vi "measure_pulse_sweep.vi"(0 "Scan settings":T1={"Start voltage (V)"=0.0, "End voltage (V)"=1.4, "Number of steps"=10, "Settling delay (ms)"=10.0, "Dual sweep"=0, "Stabilisation time (s)"=0.0, "Stabilisation mode"=0, "Stabilisation value (V or A) "=0.0, "No. of repeat scans"=2.0, "Repeat scans"=0, "Logarithmic sweep"=0, "Electrode configuration"=0, "Sweep mode"=0, "Auto settling delay"=1, "Pulse off time (ms)"=0.0, "Integration time (ms)"=1.0, "Current range"=0, "Enable display"=0, "Enable concurrent measurements"=1, "Concurrent measurements"=1} {"Concurrent measurements" items=["Volts", "Current", "Resistance", "Volt, Current", "Volts, Resistance", "Current, Resistance", "All"]; "Enable concurrent measurements" items=["False", "True"]; "Enable display" items=["False", "True"]; "Current range" items=["Auto", "1 uA", "10 uA", "100 uA", "1 mA", "10 mA", "100 mA", "1 A"]; "Integration time (ms)" min=0.2 max=200.0; "Pulse off time (ms)" min=0.0; "Auto settling delay" items=["False", "True"]; "Sweep mode" items=["Staircase", "Pulsed"]; "Electrode configuration" items=["2-wire", "4-wire"]; "Logarithmic sweep" items=["False", "True"]; "Repeat scans" items=["False", "True"]; "No. of repeat scans" min=1.0 step=1.0; "Stabilisation mode" items=["V", "I"]; "Dual sweep" items=["False", "True"]; "Settling delay (ms)" min=0.0 max=999999.9}, 7 "Area (cm^2)":dbl, 9 "VISA Refnum in":refnum<visa-resource-name>="GPIB1::26::INSTR", 11 "Filename":path, 12 "Stabilisation filename":path) -> (6 "JV Curve":cluster{dbl[], dbl[]}(graph))   [LabVIEW 2016]
uses:
  TypeDefs/settings.ctl
  <instrlib>/Keithley 24XX/Public/Data/Read (Multiple Points).vi
  <vilib>/Utility/file.llb/Write Delimited Spreadsheet (DBL).vi
  <instrlib>/Keithley 24XX/Keithley 24XX.lvlib
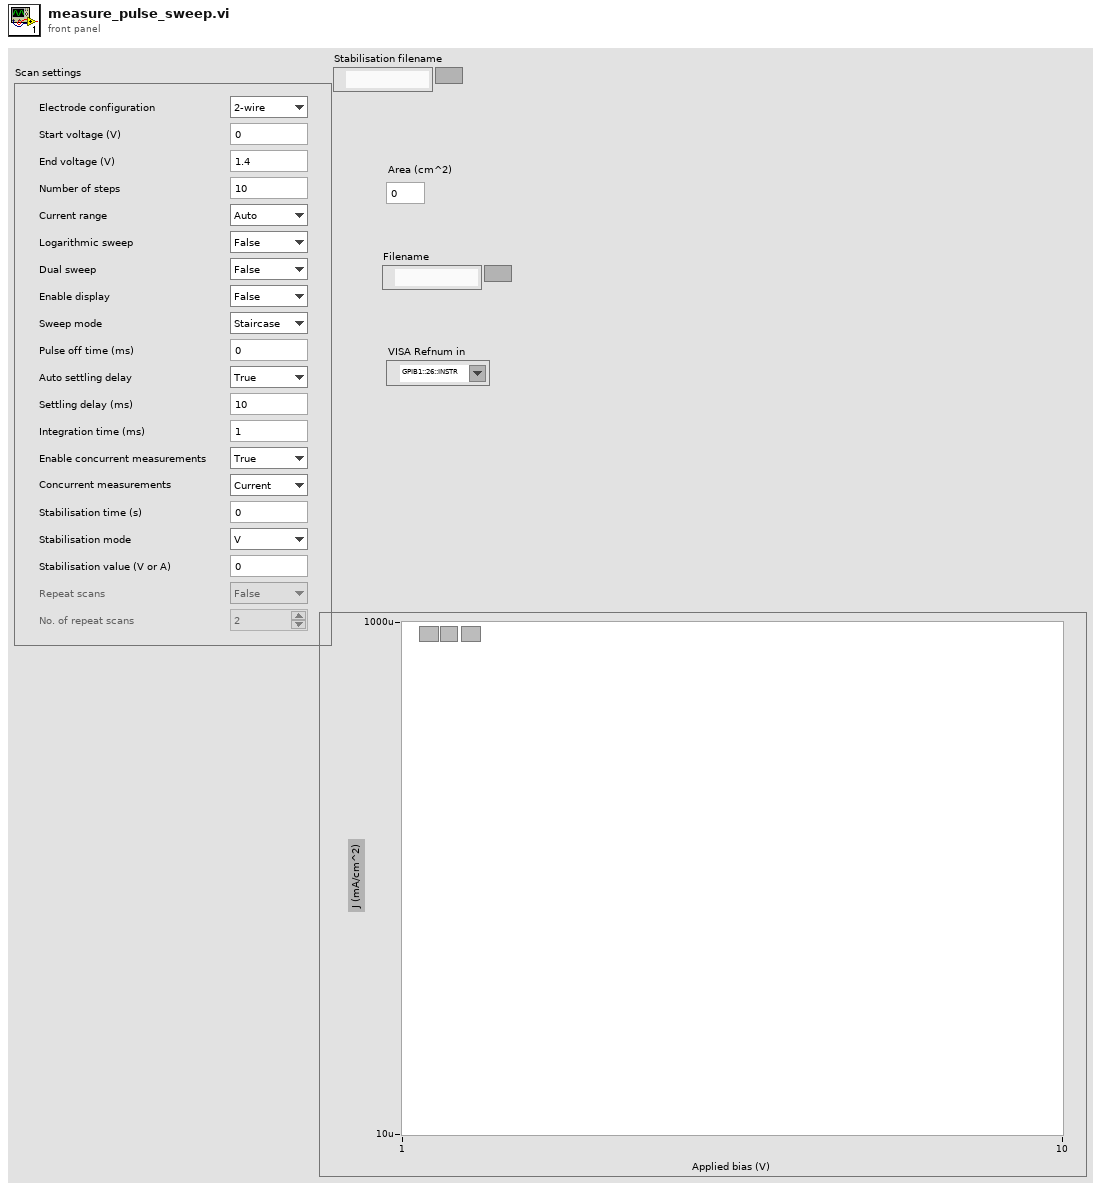
[diagram p1: front panel]
types:
  T1 = typedef "settings.ctl" = cluster{"Start voltage (V)":dbl, "End voltage (V)":dbl, "Number of steps":u32, "Settling delay (ms)":dbl, "Dual sweep":u16, "Stabilisation time (s)":dbl, "Stabilisation mode":u16, "Stabilisation value (V or A) ":dbl, "No. of repeat scans":dbl, "Repeat scans":u16, "Logarithmic sweep":u16, "Electrode configuration":u16, "Sweep mode":u16, "Auto settling delay":u16, "Pulse off time (ms)":dbl, "Integration time (ms)":dbl, "Current range":u16, "Enable display":u16, "Enable concurrent measurements":u16, "Concurrent measurements":u16}
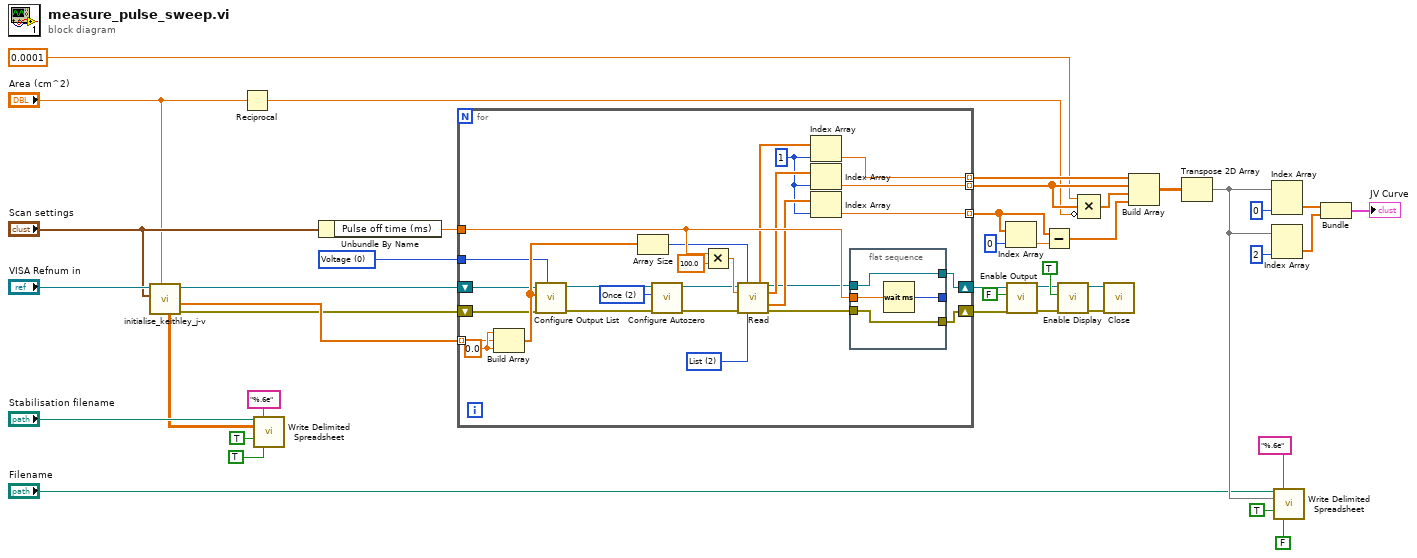
[diagram p0: block diagram]
diagram:
  w13 = u16 0 items=["Voltage", "Current"] ("Source Mode  (0: Voltage)")
  n1 = call "initialise_keithley_j-v.vi"("Area (cm^2)"="Area (cm^2)", "Scan settings"="Scan settings", "VISA Refnum in"="VISA Refnum in") -> ("error out"=w1:errorcluster, "Voltage list"=w3:dbl[], "VISA Refnum out"=w2:refnum<visa-resource-name>, "Stabilisation data"=w4:dbl[][])  [unwired: 5 in]
  n2 = Reciprocal(x="Area (cm^2)") -> (1/x=w14:dbl)
  n3 = call-poly <vilib>:"Write Delimited Spreadsheet.vi"("file path (dialog if empty)"="Stabilisation filename", "format (%.3f)"="%.6e", "2D data"=w4, "append to file? (new file:F)"=TRUE, "transpose? (no:F)"=TRUE) -> ()  [unwired: 9 in, 2 out]
  n4 = Unbundle By Name("Scan settings") -> ("Pulse off time (ms)"=w32:dbl)
  n5 = for {
    shift-right: [w68] -> w40
    shift-left: w2 -> [w48]
    shift-right: [w67] -> w39
    shift-left: w1 -> [w47]
    tunnel: w3 -> [w53] mode=indexing
    tunnel: w32 -> [w65]
    tunnel: [w62] -> w28 mode=indexing
    tunnel: [w60] -> w27 mode=indexing
    tunnel: [w57] -> w29 mode=indexing
    tunnel: w13 -> [w50]
    w46 = u16 2 items=["On", "Off", "Once"] ("Autozero  (0: On)")
    w49 = u16 2 items=["Fixed", "Sweep", "List"] ("Output Mode (0: Fixed)")
    w54 = 0.0 ("element")
    w58 = 1 ("index")
    n6 = Build Array(w54, w53, w54) -> (w52:dbl[])
    n7 = call <instrlib>:"Configure Output List.vi"("Source Mode  (0: Voltage)"=w50, "error in (no error)"=w47, "Output List"=w52, "VISA resource name"=w48) -> ("error out"=w44:errorcluster, "VISA resource name out"=w45:refnum<visa-resource-name>)  [unwired: 6 in]
    n8 = Array Size(array=w52) -> (size(s)=w51:i32)
    n9 = call <instrlib>:"Configure Autozero.vi"("error in (no error)"=w44, "Autozero  (0: On)"=w46, "VISA resource name"=w45) -> ("error out"=w42:errorcluster, "VISA resource name out"=w43:refnum<visa-resource-name>)  [unwired: 7 in]
    n10 = Multiply(x=w65, y=100.0) -> (x*y=w64:dbl)
    n11 = call-poly <instrlib>:"Read.vi"("VISA resource name"=w43, "Sample Count (1)"=w51, "Timeout (10000 ms)"=w64, "error in (no error)"=w42, "Output Mode (0: Fixed)"=w49) -> ("Voltage"=w63:sgl[], "VISA resource name out"=w55:refnum<visa-resource-name>, "Current"=w61:sgl[], "Timestamp"=w59:sgl[], "error out"=w56:errorcluster)  [unwired: 4 in, 2 out]
    n12 = Index Array(array=w63, index=w58) -> (element=w62:sgl)
    n13 = Index Array(array=w61, index=w58) -> (element=w60:sgl)
    n14 = Index Array(array=w59, index=w58) -> (element=w57:sgl)
    n15 = flat-sequence {
      tunnel: w55 -> [w72]
      tunnel: [w72] -> w68
      tunnel: w56 -> [w71]
      tunnel: [w71] -> w67
      tunnel: [w70] -> _
      tunnel: w65 -> [w69]
      frame #0 {
        n16 = Wait (ms)(milliseconds to wait=w69) -> (millisecond timer value=w70:u32)
      }
    }
  }
  n17 = Index Array(array=w29, index=0) -> (element=w30:sgl)
  n18 = call <instrlib>:"Enable Output.vi"("error in (no error)"=w39, "Enable Output (T: Enable)"=FALSE, "VISA resource name"=w40) -> ("error out"=w36:errorcluster, "VISA resource name out"=w37:refnum<visa-resource-name>)  [unwired: 7 in]
  n19 = Subtract(x=w29, y=w30) -> (x-y=w25:sgl[])
  n20 = call <instrlib>:"Enable Display.vi"("error in (no error)"=w36, "Enable Display (T: Enable)"=TRUE, "VISA resource name"=w37) -> ("error out"=w34:errorcluster, "VISA resource name out"=w35:refnum<visa-resource-name>)  [unwired: 7 in]
  n21 = Compound Arithmetic op=MULTIPLY(0.0001 ("Area (cm^2) 2"), w27, invert w14) -> (w26:dbl[])
  n22 = call <instrlib>:"Close.vi"("error in (no error)"=w34, "VISA resource name"=w35) -> ()  [unwired: 9 in, 1 out]
  n23 = Build Array(w28, w27, w26, w25) -> (w24:dbl[][])
  n24 = Transpose 2D Array(2D array=w24) -> (transposed array=w16:dbl[][])
  n25 = Index Array(array=w16, index (col)=0 ("disabled index (col)")) -> (element=w22:dbl[])  [unwired: 1 in]
  n26 = Index Array(array=w16, index (col)=2 ("disabled index (col)")) -> (element=w23:dbl[])  [unwired: 1 in]
  n27 = call-poly <vilib>:"Write Delimited Spreadsheet.vi"("file path (dialog if empty)"="Filename", "format (%.3f)"="%.6e", "2D data"=w16, "append to file? (new file:F)"=TRUE, "transpose? (no:F)"=FALSE) -> ()  [unwired: 9 in, 2 out]
  n28 = Bundle(w22, w23) -> (→"JV Curve":cluster{dbl[], dbl[]})  [unwired: 1 in]
